vi "Task Loop.vi"(8 "error in (no error)":errorcluster, 11 "EventHandlerTask in":refnum<class "EventHandlerTask.lvclass">) -> (0 "error out":errorcluster)   [LabVIEW 2020, in "Volatus.lvlib" / "EventHandlerTask.lvclass"]
uses:
  EventHandlerTask.lvclass
  EventHandlerTask.lvclass/EventHandlerTask.ctl
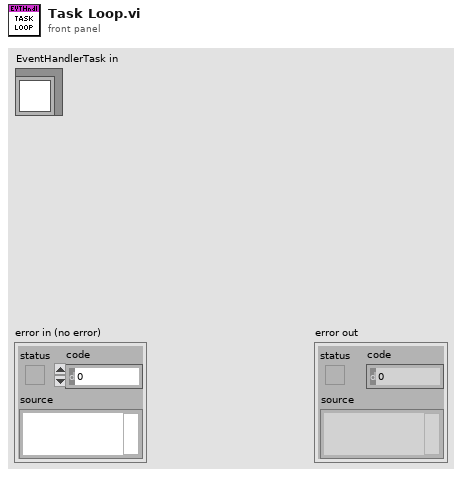
[diagram p1: front panel]
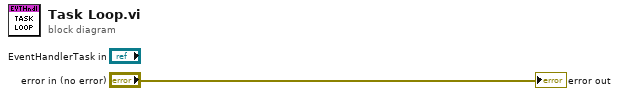
[diagram p0: block diagram]
diagram:
  "error out" <- "error in (no error)"
